vi "SetDimensions.vi"(8 "error in (no error)":errorcluster, 11 "DelayLineLS4 in":refnum<class "DLLS4.lvclass">) -> (0 "error out":errorcluster, 3 "DelayLineLS4 out":refnum<class "DLLS4.lvclass">)   [LabVIEW 2015, in "DLLS4.lvclass"]
uses:
  DLLS4.lvclass
  LS4_parameters.ctl
  DelayLine.lvclass/DelayLine.ctl
  GeneralFunctionality/GeneralFunctionality.lvclass/GeneralFunctionality.ctl
  <vilib>/Utility/error.llb/DialogType.ctl
  Config/Config.lvclass
  <vilib>/ErrorRing/Error Ring.xnode
  DelayLine.lvclass
  GeneralFunctionality/GeneralFunctionality.lvclass
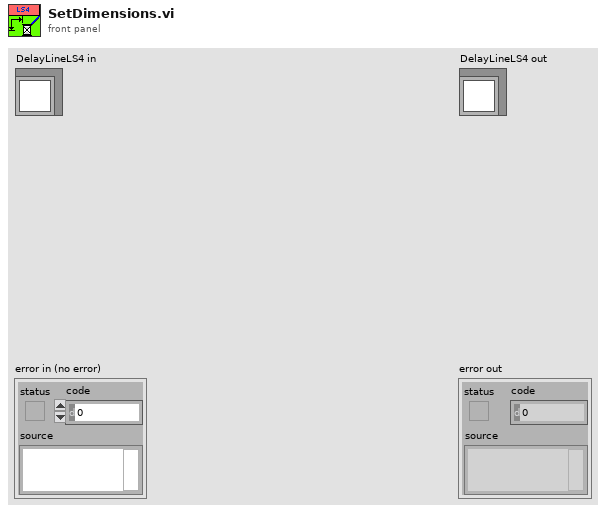
[diagram p1: front panel]
types:
  T1 = typedef "DelayLine.lvclass/LS4_parameters.ctl" = string
  T2 = typedef "DialogType.ctl" = u16
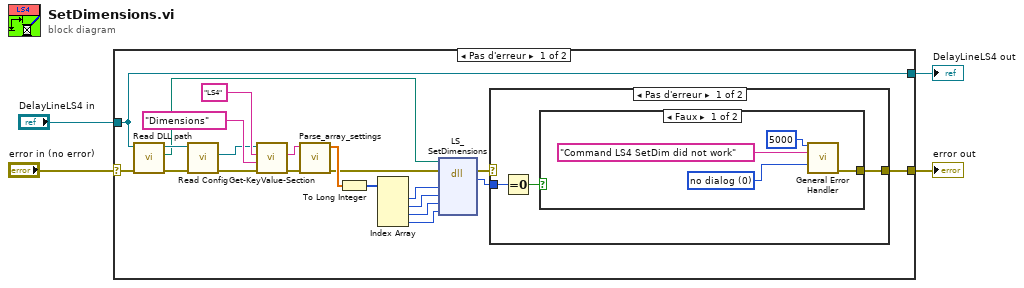
[diagram p0: block diagram]
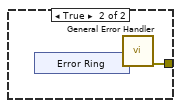
[diagram p2: hidden frame]
diagram:
  n1 = case shown="Pas d'erreur" "error in (no error)" {
    selector: "error in (no error)" -> [w14 w38]
    tunnel: [w18 w38] -> w3
    tunnel: [w17 w37] -> w1
    tunnel: "DelayLineLS4 in" -> [w17 w37]
    frame No Error {
      n2 = call "Read DLL path.vi"("error in (no error)"=w14, "DelayLine in"=w17) -> ("error out"=w16:errorcluster, "DLL path"=w13:path, "DelayLine out"=w15:refnum<class "DLLS4.lvclass">)  [unwired: 7 in]
      n3 = call "Read Config.vi"("error in (no error)"=w16, "GeneralFunctionality en entrée"=w15) -> ("error out"=w5:errorcluster, "Config.lvclass"=w8:refnum<class "Config.lvclass">)  [unwired: 7 in, 1 out]
      n4 = call-dynamic "Get-KeyValue-Section.vi"("error in (no error)"=w5, "Key"=T1 "Dimensions" ("Section"), "Section"="LS4", "Config in"=w8) -> ("error out"=w10:errorcluster, "Value"=w12:string)  [unwired: 5 in, 1 out]
      n5 = call "Parse_array_settings.vi"("error in (no error)"=w10, "Value"=w12) -> ("error out"=w6:errorcluster, "Array"=w7:sgl[])  [unwired: 8 in]
      n6 = To Long Integer(number=w7) -> (32bit integer=w19:i32[])
      n7 = Index Array(array=w19) -> (element #1=w23:i32, element #2=w22:i32, element #3=w21:i32, element #4=w20:i32)  [unwired: 4 in]
      n8 = dll-call lib="S:/TRANCON/DLL/LStep4.dll" fn="LS_SetDimensions"(path in=w13, error in=w6, "XD"=w23, "YD"=w22, "ZD"=w21, "AD"=w20) -> (error out=w24:errorcluster, "type de retour"=w25:i32)  [unwired: 5 in, 1 out]
      n9 = case shown="Pas d'erreur" w24 {
        selector: w24 -> [_ w36]
        tunnel: w25 -> [w28 _]
        tunnel: [w27 w36] -> w18
        frame No Error {
          n10 = Equal To 0?(x=w28) -> (x = 0?=w26:bool)
          n11 = case shown="Faux" w26 {
            tunnel: [w30 w33] -> w27
            frame False {
              w29 = T2 0 items=["no dialog", "OK message", "continue or stop message", "OK message + warnings", "continue/stop + warnings"] ("type of dialog (OK msg:1)")
              n12 = call <vilib>:"General Error Handler.vi"("[error code] (0)"=5000 ("code"), "[error source] (\" \")"="Command LS4 SetDim did not work" ("String to Prepend to source (\"\")"), "type of dialog (OK msg:1)"=w29) -> ("error out"=w30:errorcluster)  [unwired: 8 in, 4 out]
            }
            frame True {
              n13 = xnode "Error Ring"() -> ("sortie d'erreur"=w34:errorcluster)
              n14 = call <vilib>:"General Error Handler.vi"("error in (no error)"=w34) -> ("error out"=w33:errorcluster)  [unwired: 10 in, 4 out]
            }
          }
        }
        frame Error {
        }
      }
    }
    frame Error {
    }
  }
  "error out" <- w3
  "DelayLineLS4 out" <- w1
